vi "Replace_Saved_Coordinates1.vi"(1 "[IN] Index of staring point":i32, 2 "[IN] (X,Y,dX,dY) in Frame":dbl[](array[numeric])) -> (0 "[OUT] Replaced array":dbl[](array[numeric]))   [LabVIEW 2017]
doc: "Replacinf (labelling) of coordinates by (-1,-1) values"
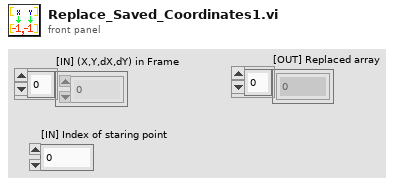
[diagram p1: front panel]
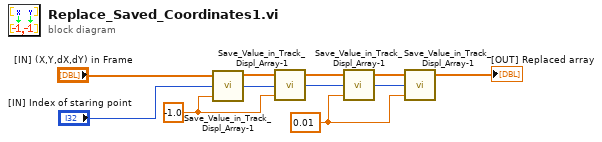
[diagram p0: block diagram]
diagram:
  w2 = 0.01 ("new element/subarray")
  w7 = -1.0 ("new element/subarray")
  n1 = call "Save_Value_in_Track_Displ_Array-1.vi"("[IN] Value"=w7, "[IN] Index"="[IN] Index of staring point", "[IN] Empty tracks\nfor points saving"="[IN] (X,Y,dX,dY) in Frame") -> ("[OUT] Index ++"=w8:i32, "[OUT Track with saved value"=w9:dbl[])  [unwired: 1 in]
  n2 = call "Save_Value_in_Track_Displ_Array-1.vi"("[IN] Value"=w7, "[IN] Index"=w8, "[IN] Empty tracks\nfor points saving"=w9) -> ("[OUT] Index ++"=w5:i32, "[OUT Track with saved value"=w6:dbl[])  [unwired: 1 in]
  n3 = call "Save_Value_in_Track_Displ_Array-1.vi"("[IN] Value"=w2, "[IN] Index"=w5, "[IN] Empty tracks\nfor points saving"=w6) -> ("[OUT] Index ++"=w3:i32, "[OUT Track with saved value"=w4:dbl[])  [unwired: 1 in]
  n4 = call "Save_Value_in_Track_Displ_Array-1.vi"("[IN] Value"=w2, "[IN] Index"=w3, "[IN] Empty tracks\nfor points saving"=w4) -> ("[OUT Track with saved value"=→"[OUT] Replaced array":dbl[])  [unwired: 1 in, 1 out]
